vi "Get Bucket ACL.vi"(8 "error in (no error)":errorcluster, 11 "Bucket in":refnum<class "Bucket.lvclass">) -> (0 "error out":errorcluster, 2 "Access Control Policy":T1, 3 "Bucket out":refnum<class "Bucket.lvclass">)   [LabVIEW 2015, in "NI_AWS_S3.lvlib" / "Bucket.lvclass"]
uses:
  Bucket.lvclass
  Access Control Policy.ctl
  User.ctl
  Grantee-Permission Pair.ctl
  Permission.ctl
  Core/HTTP Request/Request Options.ctl
  Core/HTTP Request/Name Value Pair.ctl
  Core/HTTP Request/Region handling.ctl
  Core/HTTP Request/URL formatting.ctl
  Bucket.lvclass/Bucket.ctl
  Read Name.vi
  Core/HTTP Request/HTTP Request.lvclass
  NI_AWS_S3.lvlib
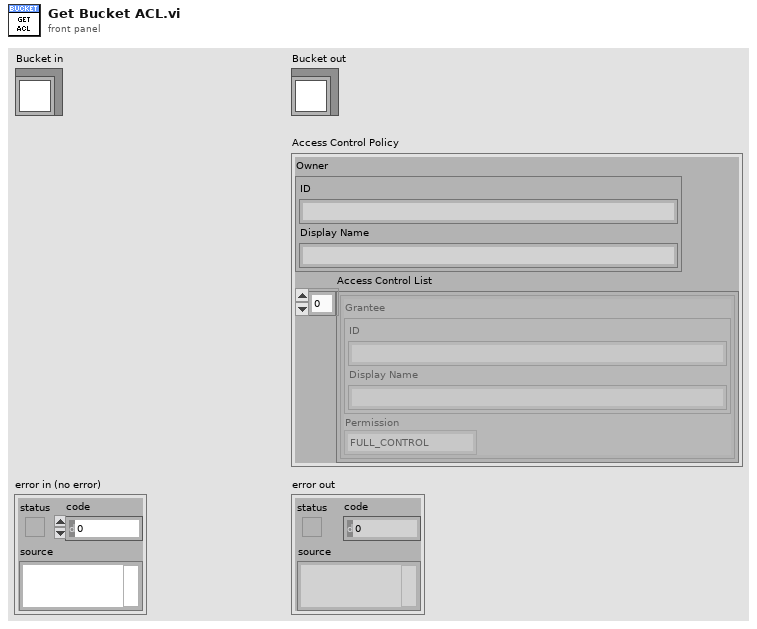
[diagram p1: front panel]
types:
  T1 = typedef "NI_AWS_S3.lvlib/Access Control Policy.ctl" = cluster{"Owner":T2, "Access Control List":T3[]}
  T2 = typedef "NI_AWS_S3.lvlib/User.ctl" = cluster{"ID":string, "Display Name":string}
  T3 = typedef "NI_AWS_S3.lvlib/Grantee-Permission Pair.ctl" = cluster{"Grantee":T2, "Permission":T4}
  T4 = typedef "NI_AWS_S3.lvlib/Permission.ctl" = enum16{"FULL_CONTROL", "WRITE", "WRITE_ACP", "READ", "READ_ACP"}
  T5 = typedef "NI_AWS_Core.lvlib/HTTP Request.lvclass/URL formatting.ctl" = enum16{"region-", "region."}
  T6 = typedef "NI_AWS_Core.lvlib/HTTP Request.lvclass/Region handling.ctl" = enum16{"use region everywhere", "use region (authentication only)", "use region (URL only)", "ignore region everwhere"}
  T7 = typedef "NI_AWS_Core.lvlib/HTTP Request.lvclass/Name Value Pair.ctl" = cluster{"name":string, "value":string}
  T8 = typedef "NI_AWS_Core.lvlib/HTTP Request.lvclass/Request Options.ctl" = cluster{"request headers":T7[], "request parameters":T7[], "request body":string, "region handling":T6, "URL formatting":T5}
  T9 = typedef "NI_AWS_Core.lvlib/HTTP Request.lvclass/Response.ctl" = cluster{"Headers":string, "Body":string}
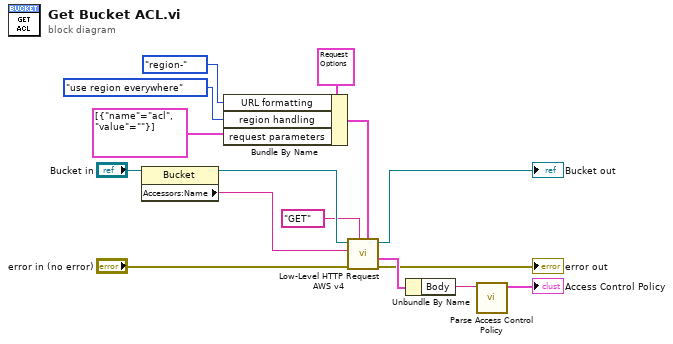
[diagram p0: block diagram]
diagram:
  n1 = property class="Bucket"(reference="Bucket in") -> (reference out=w6:refnum<class "Bucket.lvclass">, "Accessors:Name"=w7:string)  [unwired: 1 in, 1 out]
  n2 = Bundle By Name(cluster=T8 {"request headers"=[], "request parameters"=[], "request body"="", "region handling"=enum."use region everywhere", "URL formatting"=enum."region."} ("Request Options"), "URL formatting"=URL_formatting."region-", "region handling"=Region_handling."use region everywhere", "request parameters"=T7[] [{"name"="acl", "value"=""}]) -> (w4:T8)
  n3 = call "Low-Level HTTP Request AWS v4.vi"("Request Options"=w4, "HTTP-Verb"="GET", "error in (no error)"="error in (no error)", "URL Prefix"=w7, "AWS Core in"=w6) -> ("error out"=→"error out":errorcluster, "Response"=w3:T9, "AWS Core out"=→"Bucket out":refnum<class "Bucket.lvclass">)  [unwired: 3 in, 1 out]
  n4 = Unbundle By Name(w3) -> ("Body"=w10:string)
  n5 = call "Parse Access Control Policy.vi"("Body"=w10) -> ("Access Control Policy"=→"Access Control Policy":T1)  [unwired: 10 in]
